vi "oa_Remove DC Gap Reference (N Channels).vi"(0 "resampled signal":cluster{"r0":dbl, "dr":dbl, "Y":dbl[]}[](array[cluster]) {"r0" format="%.2p"; "dr" format="%.2p"; "Y" format="%.2f"}, 1 "reset?":bool=TRUE, 2 "DC ref changed?":bool=TRUE, 5 "DC gap reference [V]":dbl[](array[numeric]), 11 "error in":errorcluster, 12 "averaging type":enum16{"Linear", "Exponential"}(ring), 13 "window":T1(ring)) -> (4 "DC value out":dbl[][](array[numeric]), 8 "actual gap ref":dbl[](array[numeric]) format="%.2f", 15 "error out":errorcluster)   [LabVIEW 2017, in "SoundVib_RefDataProcess.lvlib"]
uses:
  <vilib>/addons/Sound and Vibration/Order Analysis/Referece Data Processing/SoundVib_RefDataProcess.lvlib
  <vilib>/measure/madcrms.llb/Basic Averaged DC-RMS for 1 Chan.vi
  <vilib>/measure/NI_MAPro.lvlib
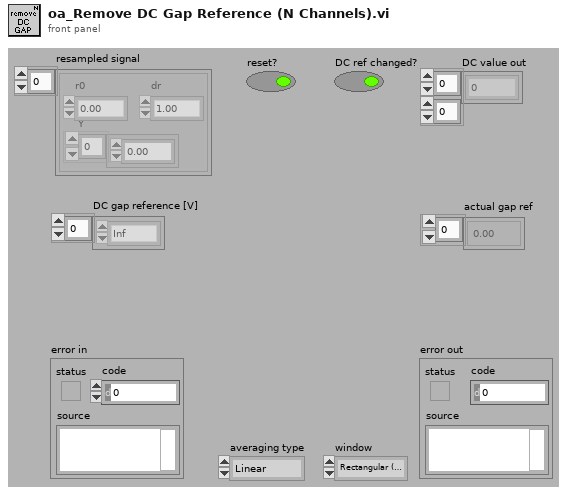
[diagram p1: front panel]
types:
  T1 = enum16{"Rectangular (none)", "Hanning", "Low side lobe"}
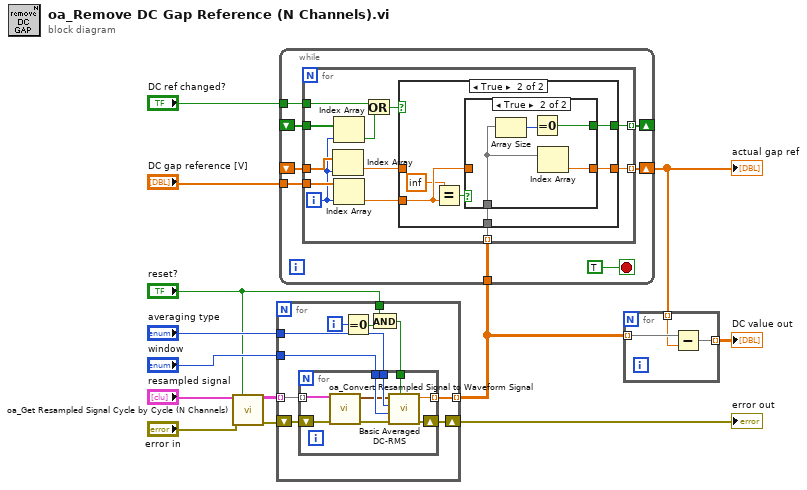
[diagram p0: block diagram]
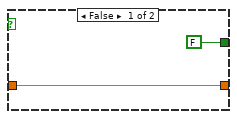
[diagram p2: hidden frame]
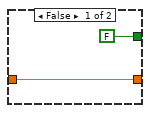
[diagram p3: hidden frame]
diagram:
  n1 = call <vilib>:"oa_Get Resampled Signal Cycle by Cycle (N Channels).vi"("resampled signal"="resampled signal", "reset?"="reset?", "error in"="error in") -> ("resampled signal out"=w5:cluster{"r0":dbl, "dr":dbl, "Y":dbl[]}[][], "error out"=w3:errorcluster)  [unwired: 11 in]
  n2 = for {
    tunnel: "window" -> [w21]
    tunnel: "averaging type" -> [w22]
    shift-right: [w23] -> w13
    shift-left: w3 -> [w14]
    tunnel: [w20] -> w8 mode=indexing
    tunnel: "reset?" -> [w17]
    tunnel: w5 -> [w15] mode=indexing
    i -> [w19]
    n3 = Equal To 0?(x=w19) -> (x = 0?=w18:bool)
    n4 = And(x=w17, y=w18) -> (x .and. y?=w16:bool)
    n5 = for {
      tunnel: w22 -> [w31]
      tunnel: w21 -> [w30]
      tunnel: [w29] -> w20 mode=indexing
      tunnel: w16 -> [w28]
      tunnel: w15 -> [w27] mode=indexing
      shift-right: [w32] -> w23
      shift-left: w14 -> [w26]
      n6 = call <vilib>:"oa_Convert Resampled Signal to Waveform Signal.vi"("resampled signal"=w27, "error in"=w26) -> ("signal in"=w25:waveform(dbl), "error out"=w24:errorcluster)  [unwired: 12 in]
      n7 = call-poly <vilib>:"Basic Averaged DC-RMS.vi"("reset"=w28, "error in (no error)"=w24, "window"=w30, "averaging type"=w31, "signal in"=w25) -> ("error out"=w32:errorcluster, "DC value"=w29:dbl)  [unwired: 3 in, 2 out]
    }
  }
  "error out" <- w13
  n8 = while {
    tunnel: "DC gap reference [V]" -> [w40]
    shift-right: [w35] -> w1
    shift-left: _ -> [w38]
    tunnel: w8 -> [w37]
    tunnel: "DC ref changed?" -> [w36]
    shift-right: [w34] -> _
    shift-left: _ -> [w33]
    stop <- TRUE stop-if-true
    n9 = for {
      tunnel: w40 -> [w51]
      tunnel: w38 -> [w47]
      tunnel: w37 -> [w52] mode=indexing
      tunnel: w36 -> [w42]
      tunnel: [w49] -> w35 mode=indexing
      tunnel: [w46] -> w34 mode=indexing
      tunnel: w33 -> [w45]
      i -> [w44]
      n10 = Index Array(array=w47, index=w44) -> (element=w48:dbl)
      n11 = Index Array(array=w45, index=w44) -> (element=w43:bool)
      n12 = Index Array(array=w51, index=w44) -> (element=w50:dbl)
      n13 = Or(x=w42, y=w43) -> (x .or. y?=w41:bool)
      n14 = case shown="True" w41 {
        tunnel: w50 -> [_ w59]
        tunnel: [w54 w56] -> w49
        tunnel: w48 -> [w54 _]
        tunnel: w52 -> [_ w60]
        tunnel: [FALSE w55] -> w46
        frame False {
        }
        frame True {
          n15 = Equal?(x=inf, y=w59) -> (x = y?=w57:bool)
          n16 = case shown="True" w57 {
            tunnel: [w62 w66] -> w56
            tunnel: w59 -> [w62 _]
            tunnel: w60 -> [_ w65]
            tunnel: [FALSE w63] -> w55
            frame False {
            }
            frame True {
              n17 = Array Size(array=w65) -> (size(s)=w64:i32)
              n18 = Equal To 0?(x=w64) -> (x = 0?=w63:bool)
              n19 = Index Array(array=w65) -> (element=w66:dbl)  [unwired: 1 in]
            }
          }
        }
      }
    }
  }
  "actual gap ref" <- w1
  n20 = for {
    tunnel: w8 -> [w69] mode=indexing
    tunnel: w1 -> [w68] mode=indexing
    tunnel: [w67] -> w7 mode=indexing
    n21 = Subtract(x=w69, y=w68) -> (x-y=w67:dbl[])
  }
  "DC value out" <- w7
